vi "GetType.vi"(8 "error in (no error)":errorcluster, 11 "Force Move LogFiles Msg":refnum<class "Force Move LogFiles Msg.lvclass">) -> (0 "error out":errorcluster, 2 "Data Sample":variant, 3 "Force Move LogFiles Msg":refnum<class "Force Move LogFiles Msg.lvclass">)   [LabVIEW 2015, in "KIT-QVA.lvlib" / "Force Move LogFiles Msg.lvclass"]
uses:
  Force Move LogFiles Msg.lvclass
  Force Move LogFiles Msg.lvclass/Force Move LogFiles Msg.ctl
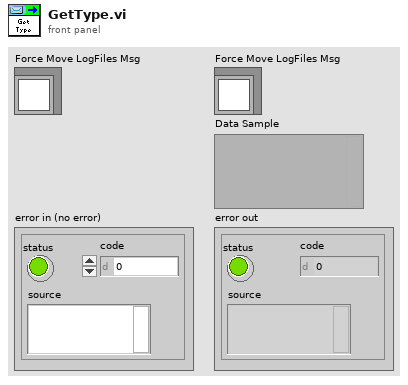
[diagram p1: front panel]
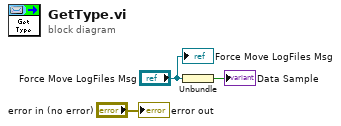
[diagram p0: block diagram]
diagram:
  n1 = Unbundle("Force Move LogFiles Msg") -> (→"Data Sample":bool)
  "error out" <- "error in (no error)"
  "Force Move LogFiles Msg" <- "Force Move LogFiles Msg"
